vi "MakePrefix.vi"(8 "TempPoint":i32, 9 "TempCycleNo":i32, 10 "FolderPrefix":string, 11 "TopFolderPath":path=path "C:/Users/dpl/OneDrive - Aberystwyth University/Documents/LabVIEW Data/TestExecutive/TestData") -> (2 "Prefix":string, 3 "TestFolderPath":path)   [LabVIEW 2024]
uses:
  <userlib>/_OpenG.lib/file/file.llb/openg_file.lvlib
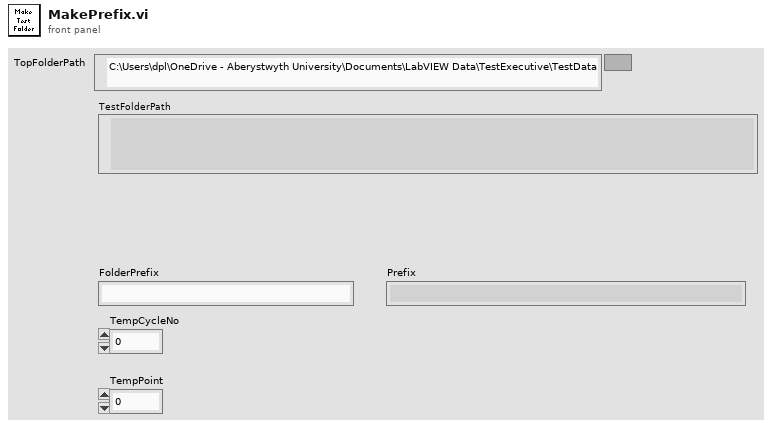
[diagram p1: front panel]
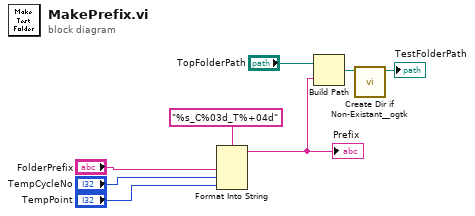
[diagram p0: block diagram]
diagram:
  n1 = Format Into String(format string="%s_C%03d_T%+04d", "FolderPrefix", "TempCycleNo", "TempPoint") -> (resulting string=w1:string)  [unwired: 2 in, 1 out]
  "Prefix" <- w1
  n2 = Build Path(base path="TopFolderPath", name or relative path=w1) -> (appended path=w4:path)
  n3 = call <userlib>:"Create Dir if Non-Existant__ogtk.vi"("Directory Path"=w4) -> ("dup Directory Path"=→"TestFolderPath":path)  [unwired: 8 in, 2 out]
